vi "GOOPUtil_IsValidReference.vi"(0 "LabVIEW Object":refnum<class>, 5 "error in (no error)":errorcluster) -> (14 "Not a refnum?":bool, 15 "Class Name":string, 19 "error out":errorcluster)   [LabVIEW 2012, in "GOOPUtility.lvlib"]
doc: "Checks if a reference contains a valid GOOP reference.\n\nThis is a collection of generic GOOP utility VIs. Please notice that it is important that the frontpanel of the Create, Destroy and GetObjectStatus is not removed when building an application."
uses:
  <vilib>/addons/GOOPUtility/GOOPUtility.lvlib
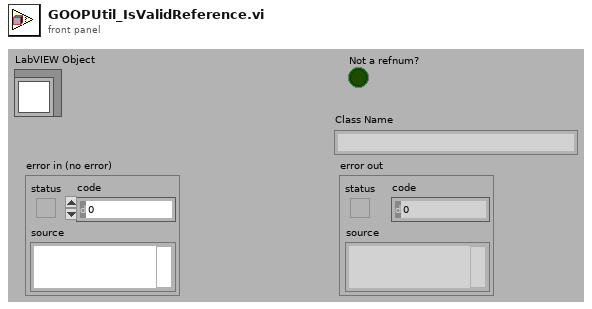
[diagram p1: front panel]
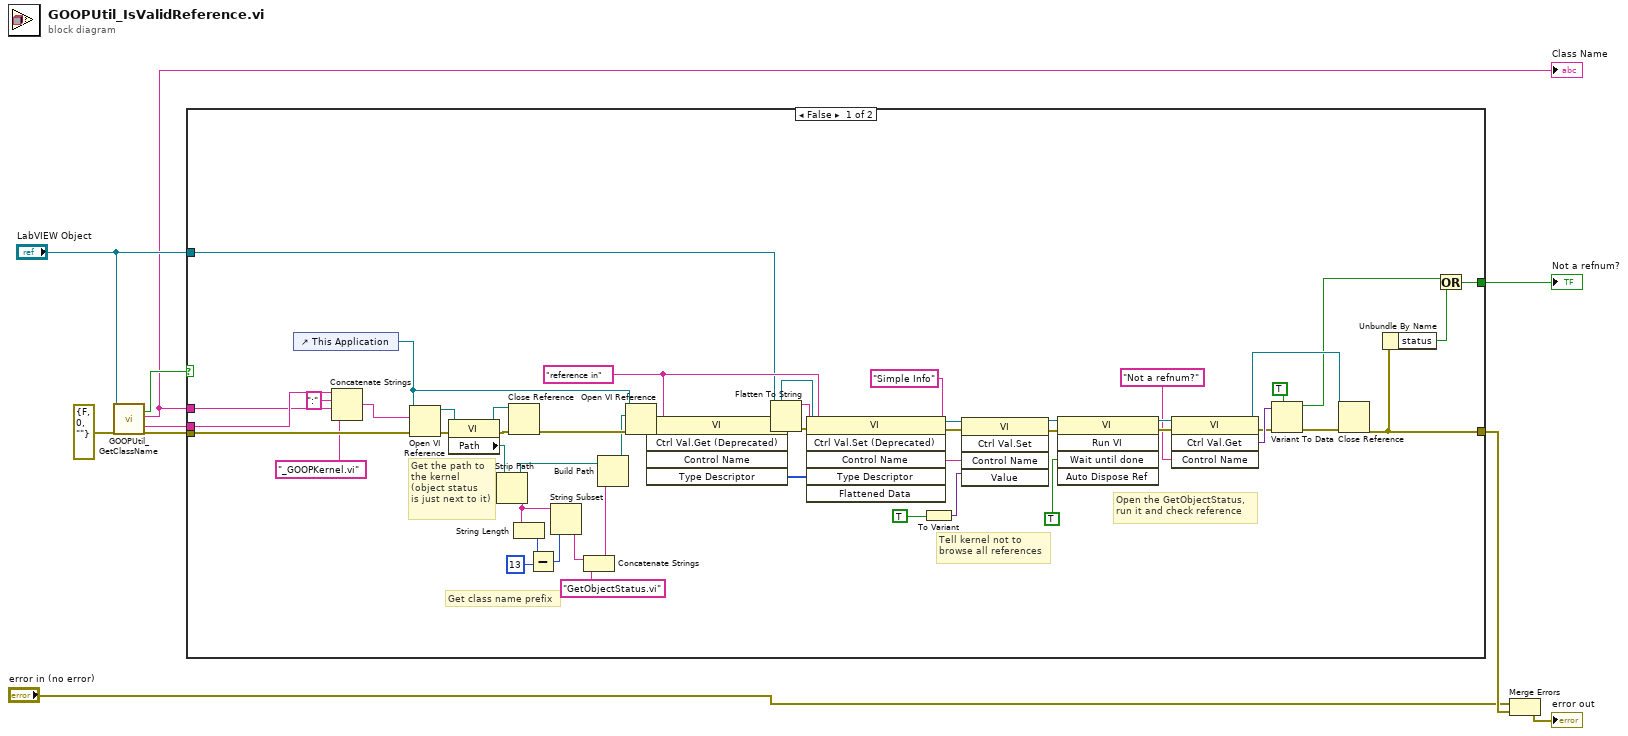
[diagram p0: block diagram]
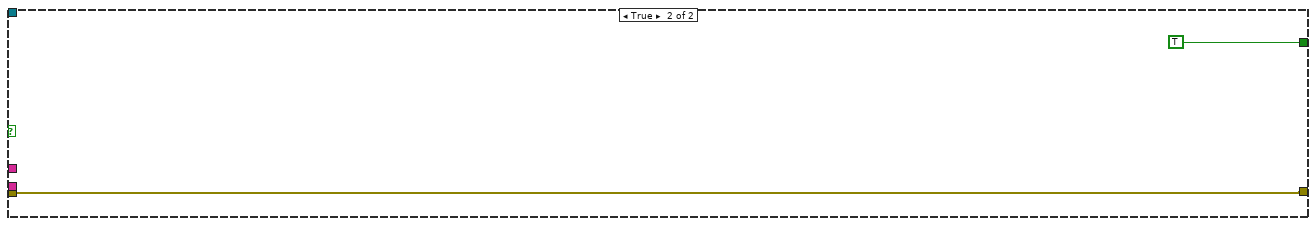
[diagram p2: hidden frame]
diagram:
  n1 = call <vilib>:"GOOPUtil_GetClassName.vi"("LabVIEW Object"="LabVIEW Object", "error in (no error)"=errorcluster {"status"=FALSE, "code"=0, "source"=""}) -> ("IsEmptyObject?"=w9:bool, "Class Name"=w1:string, "Full Class Name"=w2:string, "error out"=w8:errorcluster)  [unwired: 13 in, 1 out]
  "Class Name" <- w1
  n2 = case shown="False" w9 {
    tunnel: "LabVIEW Object" -> [w37 _]
    tunnel: w8 -> [w17 w62]
    tunnel: [w31 TRUE] -> w6
    tunnel: [w18 w62] -> w4
    tunnel: w2 -> [w16 _]
    tunnel: w1 -> [w14 _]
    frame False {
      w42 = "reference in" ("Control Name")
      # "Tell kernel not to\nbrowse all references"
      # "Open the GetObjectStatus,\nrun it and check reference"
      # "Get the path to\nthe kernel\n(object status\nis just next to it)"
      # "Get class name prefix"
      n3 = control-ref of="This Application"() -> (w12:refnum<vi>)
      n4 = Concatenate Strings(w16, ":" ("string"), w14, "_GOOPKernel.vi") -> (w11:string)
      n5 = Open VI Reference(application reference (local)=w12, vi path=w11, error in (no error)=w17) -> (vi reference=w60:refnum<vi>, error out=w61:errorcluster)  [unwired: 3 in]
      n6 = property class="VI"(reference=w60, error in=w61) -> (reference out=w58:refnum<vi>, error out=w59:errorcluster, "Path"=w56:path)
      n7 = Strip Path(path=w56) -> (stripped path=w46:path, name=w52:string)
      n8 = Close Reference(reference=w58, error in (no error)=w59) -> (error out=w57:errorcluster)
      n9 = String Length(string=w52) -> (length=w55:i32)
      n10 = Subtract(x=w55, y=13) -> (x-y=w53:i32)
      n11 = String Subset(string=w52, length (rest)=w53) -> (substring=w47:string)  [unwired: 1 in]
      n12 = Concatenate Strings(w47, "GetObjectStatus.vi") -> (w50:string)
      n13 = Build Path(base path=w46, name or relative path=w50) -> (appended path=w49:path)
      n14 = Open VI Reference(application reference (local)=w12, vi path=w49, error in (no error)=w57) -> (vi reference=w44:refnum<vi>, error out=w45:errorcluster)  [unwired: 3 in]
      n15 = invoke class="VI" method="Ctrl Val.Get (Deprecated)"(reference=w44, error in=w45, "Control Name"=w42) -> (reference out=w43:refnum<vi>, error out=w40:errorcluster, "Type Descriptor"=w41:i16[])  [unwired: 2 in, 2 out]
      n16 = Flatten To String(anything=w37, error in (no error)=w40) -> (data string=w38:string, error out=w39:errorcluster)  [unwired: 2 in, 1 out]
      n17 = invoke class="VI" method="Ctrl Val.Set (Deprecated)"(reference=w43, error in=w39, "Control Name"=w42, "Type Descriptor"=w41, "Flattened Data"=w38) -> (reference out=w29:refnum<vi>, error out=w30:errorcluster)  [unwired: 1 in, 4 out]
      n18 = To Variant(anything=TRUE ("Wait Until Done")) -> (Variant=w19:variant)
      n19 = invoke class="VI" method="Ctrl Val.Set"(reference=w29, error in=w30, "Control Name"="Simple Info", "Value"=w19) -> (reference out=w27:refnum<vi>, error out=w28:errorcluster)  [unwired: 1 in, 3 out]
      n20 = invoke class="VI" method="Run VI"(reference=w27, error in=w28, "Wait until done"=TRUE ("Wait Until Done")) -> (reference out=w35:refnum<vi>, error out=w36:errorcluster)  [unwired: 2 in, 3 out]
      n21 = invoke class="VI" method="Ctrl Val.Get"(reference=w35, error in=w36, "Control Name"="Not a refnum?") -> (reference out=w33:refnum<vi>, error out=w24:errorcluster, "Get Control Value Variant"=w25:variant)  [unwired: 1 in, 1 out]
      n22 = Variant To Data(error in=w24, type=TRUE, Variant=w25) -> (data=w21:bool, error out=w23:errorcluster)
      n23 = Close Reference(reference=w33, error in (no error)=w23) -> (error out=w18:errorcluster)
      n24 = Unbundle By Name(w18) -> ("status"=w32:bool)
      n25 = Or(x=w21, y=w32) -> (x .or. y?=w31:bool)
    }
    frame True {
    }
  }
  "Not a refnum?" <- w6
  n26 = Merge Errors("error in (no error)", w4) -> (→"error out":errorcluster)
